vi "Configure Limit.vi"(0 "VISA resource name":refnum<visa-resource-name>, 5 "error in (no error)":errorcluster, 6 "State":bool, 9 "Lower Limit":dbl, 11 "Upper Limit":dbl) -> (14 "VISA resource name out":refnum<visa-resource-name>, 19 "error out":errorcluster)   [LabVIEW 2020, in "Keithley 2100 Series.lvlib"]
doc: "Definition:\nThe limits testing operation allows user to adjust a maximal and a minimal limit values. The multimeter beeps and an “HI” or “LO” message will be shown when the reading exceeds the upper or lower limit respectively. Users can specify the limit values and the values are stored\nin a volatile memory. The default values for both upper and lower limits are “0”. This function is available to all except continuity and diode measurements.\n\nRemote Interface Operation:\n\nUse the following commands to enable the limits function or to set the limits:\n\nCALCulate:FUNCtion LIMit\nCALCulate:STATe {OFF|ON}\nCALCulate:STATe?\nCALCulate:LIMit:LOWer {<value>|MINimum|MAXimum}\nCALCulate:LIMit:UPPer {<value>|MINimum|MAXimum}"
uses:
  Keithley 2100 Series.lvlib
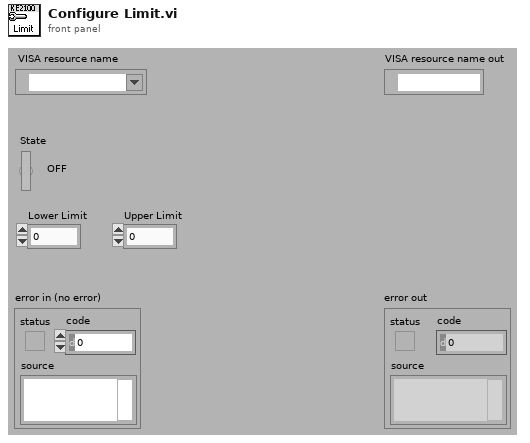
[diagram p1: front panel]
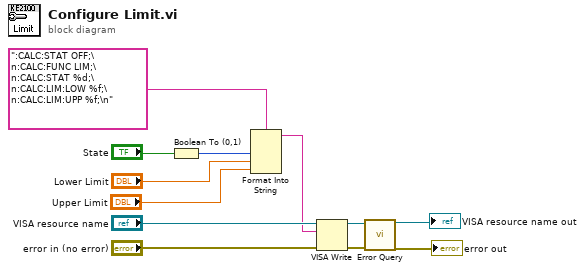
[diagram p0: block diagram]
diagram:
  n1 = Boolean To (0,1)(Boolean="State") -> (0, 1=w5:i16)
  n2 = Format Into String(format string=":CALC:STAT OFF;\n:CALC:FUNC LIM;\n:CALC:STAT %d;\n:CALC:LIM:LOW %f;\n:CALC:LIM:UPP %f;\n", w5, "Lower Limit", "Upper Limit") -> (resulting string=w6:string)  [unwired: 2 in, 1 out]
  n3 = VISA Write(VISA resource name="VISA resource name", write buffer=w6, error in (no error)="error in (no error)") -> (VISA resource name out=w11:refnum<visa-resource-name>, error out=w12:errorcluster)  [unwired: 1 out]
  n4 = call "Error Query.vi"("VISA resource name"=w11, "error in (no error)"=w12) -> ("VISA resource name out"=→"VISA resource name out":refnum<visa-resource-name>, "error out"=→"error out":errorcluster)  [unwired: 14 in, 2 out]
